vi "ASI Get Control Value.vi"(7 "pbAuto":i32, 9 "plValue":i32, 10 "ControlType":i32, 11 "iCameraID":i32) -> (1 "plValue out":i32, 3 "function return":i32, 5 "pbAuto out":i32)   [LabVIEW 2012, in "ASICamera2_no_err.lvlib"]
doc: "ASICAMERA_API ASI_ERROR_CODE ASIGetControlValue(int iCameraID, ASI_CONTROL_TYPE ControlType, long *plValue, ASI_BOOL *pbAuto);"
uses:
  <userlib>/ASICamera2_no_err/ASICamera2_no_err.lvlib
  ASICamera2.dll
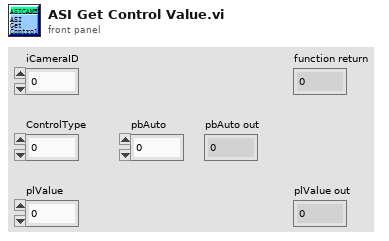
[diagram p1: front panel]
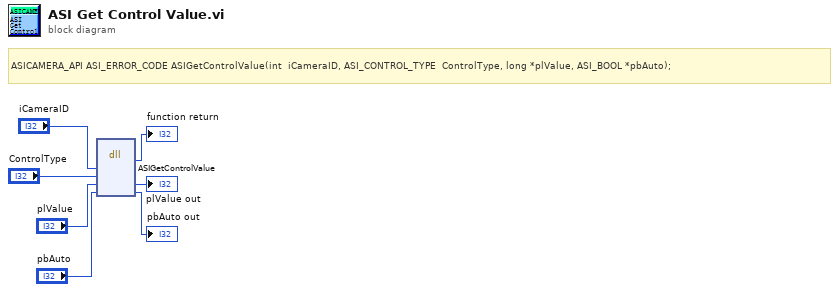
[diagram p0: block diagram]
diagram:
  # "ASICAMERA_API ASI_ERROR_CODE ASIGetControlValue(int  iCameraID, ASI_CONTROL_TYPE  ControlType, long *plValue, ASI_BOOL *pbAuto);"
  n1 = dll-call lib="ASICamera2.*" fn="ASIGetControlValue"("iCameraID"="iCameraID", "ControlType"="ControlType", "plValue"="plValue", "pbAuto"="pbAuto") -> (→"function return":i32, "plValue"=→"plValue out":i32, "pbAuto"=→"pbAuto out":i32)  [unwired: 5 in, 2 out]
